vi "Create Shared Resources.vi"(8 "error in":errorcluster, 10 "custom device ref":T1=18446744073709551615 format="%.0x", 11 "shared resources factory in":refnum<class "Shared Resources Factory.lvclass">) -> (0 "error out":errorcluster, 2 "shared resources":refnum<class "Shared Resources.lvclass">, 3 "shared resources factory out":refnum<class "Shared Resources Factory.lvclass">)   [LabVIEW 2020, in "AIM ARINC 429 Engine.lvlib" / "Implementation.lvlib" / "Shared Resources Factory.lvclass"]
uses:
  Shared Resources Factory.lvclass
  Scripting/AIM/AIM ARINC 429 Scripting.lvlib
  Shared Resources/Shared Resources.lvclass
  Custom Device/Logging Configuration.ctl
  Custom Device/Custom Device.lvlib
  Shared/Data Word Format.ctl
  C:/Users/nitest/Documents/LabVIEW Data/AIM ARINC 429/Source/Custom Device Support/Engine/Implementation/Shared Resources/Shared Resources.lvclass
  C:/Users/nitest/Documents/LabVIEW Data/AIM ARINC 429/Source/Custom Device Support/Engine/Interfaces/Shared Resources/Shared Resources.lvclass
  <vilib>/NI VeriStand/Custom Device API/Custom Device Item Ref.ctl
  <vilib>/NI VeriStand/Custom Device API/Custom Device API.lvlib
  Interfaces/Shared Resources/Shared Resources.lvclass
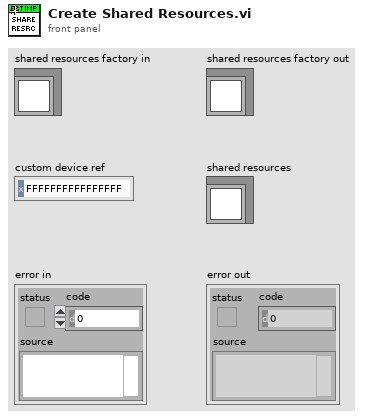
[diagram p1: front panel]
types:
  T1 = typedef "Custom Device API.lvlib/Custom Device Item Ref.ctl" = u64
  T2 = typedef "AIM ARINC 429 Engine.lvlib/Custom Device.lvlib/Logging Configuration.ctl" = cluster{"configured":bool, "directory":string, "file name":string, "timestamp file name":bool, "data word format":T3}
  T3 = typedef "Data Word Format.ctl" = string
  T4 = typedef "Device Parameters.ctl" = cluster{"initialization method":T5, "card number":i32, "PXI slot number":i32, "core number":i32}
  T5 = typedef "Initialization Method.ctl" = enum16{"PXI Slot Number", "Card Number"}
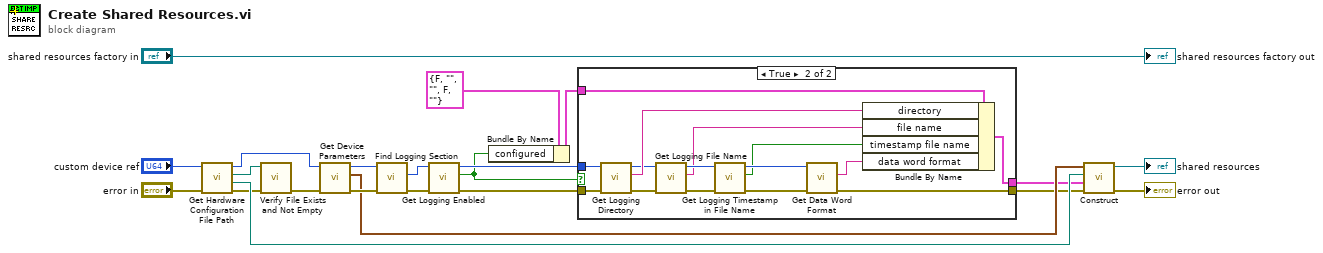
[diagram p0: block diagram]
diagram:
  n1 = call "Get Hardware Configuration File Path.vi"("error in"="error in", "Ballard ARINC 429 custom device in"="custom device ref") -> ("error out"=w16:errorcluster, "RT destination"=w19:path, "hardware configuration file path"=w17:path, "Ballard ARINC 429 custom device out"=w11:T1)  [unwired: 6 in]
  n2 = call "Verify File Exists and Not Empty.vi"("error in"=w16, "path"=w17) -> ("error out"=w14:errorcluster)  [unwired: 9 in]
  n3 = call "Get Device Parameters.vi"("error in"=w14, "Ballard ARINC 429 custom device in"=w11) -> ("error out"=w22:errorcluster, "device parameters"=w20:T4, "Ballard ARINC 429 custom device out"=w9:T1)  [unwired: 7 in]
  n4 = call "Find Logging Section.vi"("error in"=w22, "Ballard ARINC 429 custom device in"=w9) -> ("error out"=w5:errorcluster, "logging"=w8:T1)  [unwired: 7 in, 1 out]
  n5 = call "Get Logging Enabled.vi"("error in"=w5, "logging in"=w8) -> ("error out"=w4:errorcluster, "logging enabled"=w1:bool, "logging out"=w6:T1)  [unwired: 7 in]
  n6 = Bundle By Name(cluster=T2 {"configured"=FALSE, "directory"="", "file name"="", "timestamp file name"=FALSE, "data word format"=""} ("logging configuration"), "configured"=w1) -> (w2:T2)
  n7 = case shown="True" w1 {
    tunnel: [w24 w33] -> w10
    tunnel: [w23 w37] -> w7
    tunnel: w6 -> [_ w36]
    tunnel: w4 -> [w24 w35]
    tunnel: w2 -> [w23 w34]
    frame False {
    }
    frame True {
      n8 = call "Get Logging Directory.vi"("error in"=w35, "logging in"=w36) -> ("error out"=w39:errorcluster, "directory"=w38:string, "logging out"=w29:T1)  [unwired: 7 in]
      n9 = call "Get Logging File Name.vi"("error in"=w39, "logging in"=w29) -> ("error out"=w31:errorcluster, "file name"=w26:string, "logging out"=w28:T1)  [unwired: 7 in]
      n10 = call "Get Logging Timestamp in File Name.vi"("error in"=w31, "logging in"=w28) -> ("error out"=w30:errorcluster, "timestamp in file name"=w25:bool, "logging out"=w27:T1)  [unwired: 7 in]
      n11 = call "Get Data Word Format.vi"("error in"=w30, "logging in"=w27) -> ("error out"=w33:errorcluster, "data word format"=w32:T3)  [unwired: 7 in, 1 out]
      n12 = Bundle By Name(cluster=w34, "directory"=w38, "file name"=w26, "timestamp file name"=w25, "data word format"=w32) -> (w37:T2)
    }
  }
  n13 = call "Construct.vi"("error in"=w10, "logging configuration"=w7, "hardware configuration file on target"=w19, "device parameters"=w20) -> ("error out"=→"error out":errorcluster, "Ballard ARINC-429 shared resources out"=→"shared resources":refnum<class "Shared Resources.lvclass">)  [unwired: 6 in]
  "shared resources factory out" <- "shared resources factory in"
